vi "AssertSubpanelVI.vi"(0 "VI Reference In":refnum<vi>, 1 "Test Label":string, 2 "delimiter (>>)":string=">>", 3 "Assert Only? (F)":bool, 5 "Control Path":string, 7 "VI Name":string, 11 "Error In":errorcluster, 12 "Assert Interval(10 ms)":u32=10, 13 "Timeout(5 sec)":dbl=5.0) -> (4 "VI Reference Out":refnum<vi>, 6 "Asserted Value":string, 15 "Error Out":errorcluster)   [LabVIEW 2016, in "Drona.lvlib" / "AssertControlValue.lvlib" / "AssertSubpanel.lvlib"]
doc: "Asserts if the Inserted VI in Subpanel is the same VI as given by VI name input.\nThe input control name is given as a string , incase of path, use delimiters inbetween the path."
uses:
  AssertSubpanel.lvlib
  Get/GetControlRef/GetControlRefByPath.vi
  <vilib>/addons/_JKI Toolkits/Caraya/classes/Assert/Assert Equal Value_Variant.vi
  <vilib>/addons/_JKI Toolkits/Caraya/classes/Assert/Assert.lvclass
  Get/GetControlRef/GetControlRef.lvlib
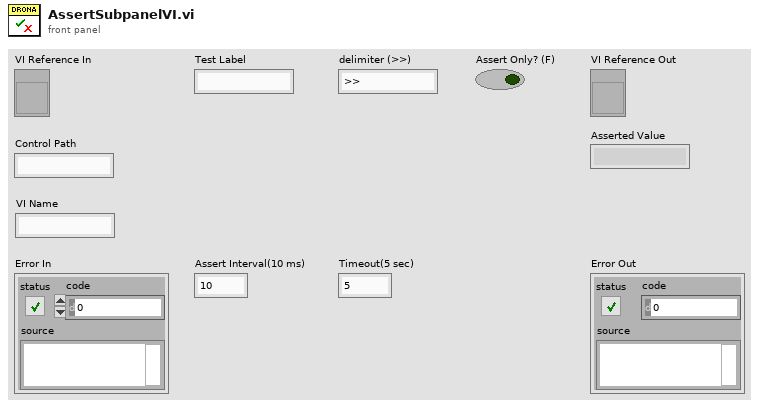
[diagram p1: front panel]
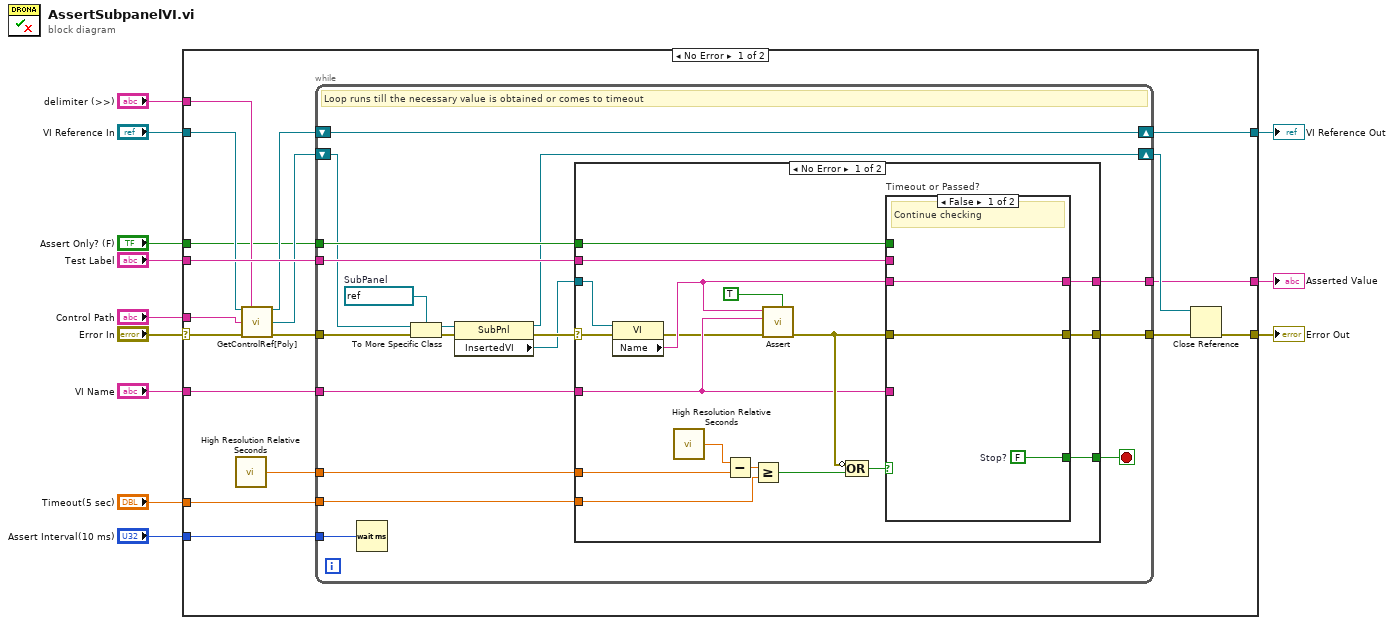
[diagram p0: block diagram]
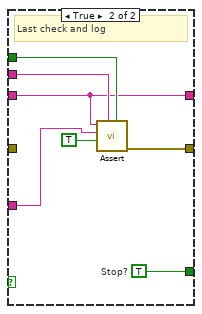
[diagram p2: hidden frame]
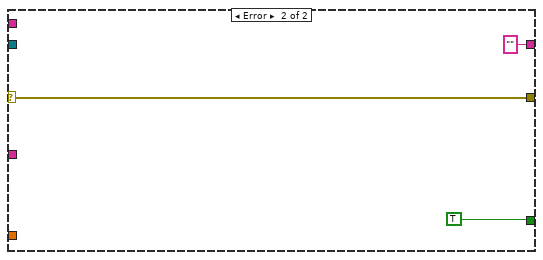
[diagram p3: hidden frame]
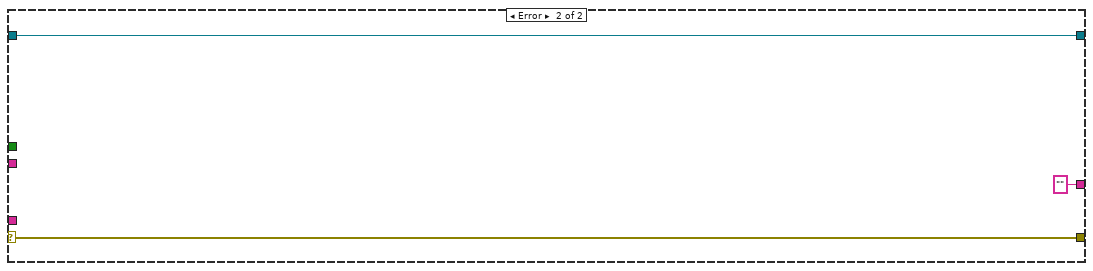
[diagram p4: hidden frame]
diagram:
  n1 = case shown="No Error" "Error In" {
    selector: "Error In" -> [w26 w82]
    tunnel: "Timeout(5 sec)" -> [w30 _]
    tunnel: [w29 w81] -> w11
    tunnel: [w19 w82] -> w10
    tunnel: "Assert Interval(10 ms)" -> [w28 _]
    tunnel: "Test Label" -> [w27 _]
    tunnel: "VI Reference In" -> [w25 w81]
    tunnel: "Control Path" -> [w24 _]
    tunnel: "delimiter (>>)" -> [w18 _]
    tunnel: "Assert Only? (F)" -> [w17 _]
    tunnel: "VI Name" -> [w16 _]
    tunnel: [w13 "" ("Name")] -> w1
    frame No Error {
      n2 = call <vilib>:"High Resolution Relative Seconds.vi"() -> ("relative seconds"=w23:dbl)
      n3 = call-poly "GetControlRef[Poly].vi"("VI Reference In"=w25, "delimiter (>>)"=w18, "Control Path"=w24, "error In"=w26) -> ("VI Reference Out"=w21:refnum<vi>, "Ctl Refnum"=w20:refnum<vi>, "error out"=w22:errorcluster)  [unwired: 9 in]
      n4 = while {
        tunnel: w30 -> [w47]
        tunnel: w23 -> [w48]
        tunnel: w22 -> [w43]
        tunnel: [w32] -> w15
        tunnel: w28 -> [w44]
        tunnel: w27 -> [w41]
        shift-right: [w42] -> w29
        shift-left: w21 -> [w42]
        tunnel: w17 -> [w40]
        tunnel: w16 -> [w38]
        shift-right: [w33] -> w14
        shift-left: w20 -> [w35]
        tunnel: [w31] -> w13
        stop <- w46 stop-if-true
        w36 = refnum<vi> refnum  # SubPanel
        # "Loop runs till the necessary value is obtained or comes to timeout"
        n5 = Wait (ms)(milliseconds to wait=w44) -> ()  [unwired: 1 out]
        n6 = To More Specific Class(target class=w36, reference=w35, error in=w43) -> (specific class reference=w34:refnum<vi>, error out=w37:errorcluster)
        n7 = property class="SubPnl"(reference=w34, error in=w37) -> (reference out=w33:refnum<vi>, error out=w45:errorcluster, "InsertedVI"=w39:refnum<vi>)
        n8 = case shown="No Error" w45 {
          selector: w45 -> [w51 w79]
          tunnel: w48 -> [w66 _]
          tunnel: w47 -> [w63 _]
          tunnel: [w56 TRUE] -> w46
          tunnel: [w57 w79] -> w32
          tunnel: w39 -> [w53 _]
          tunnel: w41 -> [w62 _]
          tunnel: w40 -> [w55 _]
          tunnel: w38 -> [w54 _]
          tunnel: [w49 "" ("Name")] -> w31
          frame No Error {
            n9 = property class="VI"(reference=w53, error in=w51) -> (error out=w50:errorcluster, "Name"=w52:string)  [unwired: 1 out]
            n10 = call <vilib>:"High Resolution Relative Seconds.vi"() -> ("relative seconds"=w65:dbl)
            n11 = Subtract(x=w65, y=w66) -> (x-y=w64:dbl)
            n12 = Greater Or Equal?(x=w64, y=w63) -> (x >= y?=w61:bool)
            n13 = call-poly <vilib>:"Assert.vi"("Assert Only? (F)"=TRUE, "error in (no error)"=w50, "Y"=w54, "X"=w52) -> ("error out"=w60:errorcluster)  [unwired: 6 in, 1 out]
            n14 = Compound Arithmetic op=OR(invert w60, w61) -> (w59:bool)
            n15 = case "Timeout or Passed?" shown="False" w59 {
              tunnel: w60 -> [w69 _]
              tunnel: w52 -> [w67 w70]
              tunnel: w62 -> [_ w76]
              tunnel: [w69 w71] -> w57
              tunnel: [w68 w75] -> w56
              tunnel: w55 -> [_ w73]
              tunnel: w54 -> [_ w72]
              tunnel: [w67 w70] -> w49
              frame False {
                w68 = FALSE  # Stop?
                # "Continue checking"
              }
              frame True {
                w75 = TRUE  # Stop?
                # "Last check and log"
                n16 = call-poly <vilib>:"Assert.vi"("Assert Only? (F)"=w73, "Label"=w76, "Register with caller test (F)"=TRUE, "Y"=w72, "X"=w70) -> ("error out"=w71:errorcluster)  [unwired: 5 in, 1 out]
              }
            }
          }
          frame Error {
          }
        }
      }
      n17 = Close Reference(reference=w14, error in (no error)=w15) -> (error out=w19:errorcluster)
    }
    frame Error {
    }
  }
  "Error Out" <- w10
  "VI Reference Out" <- w11
  "Asserted Value" <- w1
